vi "Str To Colorbox.vi"(1 "String":string) -> (0 "Color Box":u32(colorbox))   [LabVIEW 2017]
doc: "Converts a colour string into the 32-bit RGB value that a LabVIEW colour box control displays."
uses:
  _openG/_reuse_openG.lvlib
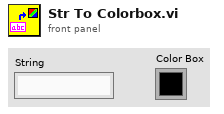
[diagram p1: front panel]
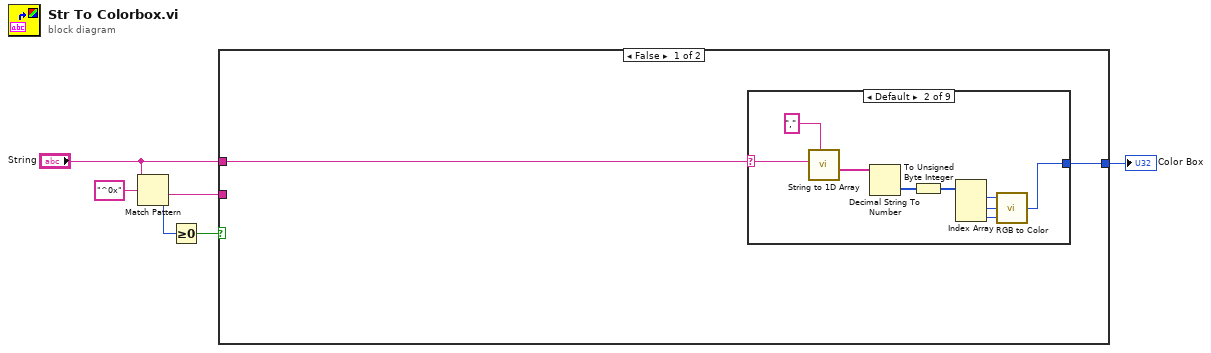
[diagram p0: block diagram]
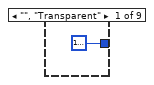
[diagram p2: hidden frame]
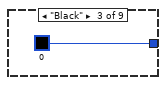
[diagram p3: hidden frame]
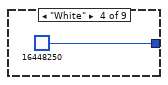
[diagram p4: hidden frame]
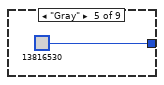
[diagram p5: hidden frame]
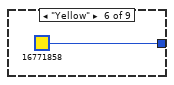
[diagram p6: hidden frame]
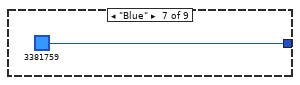
[diagram p7: hidden frame]
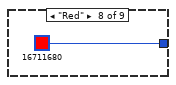
[diagram p8: hidden frame]
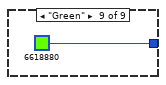
[diagram p9: hidden frame]
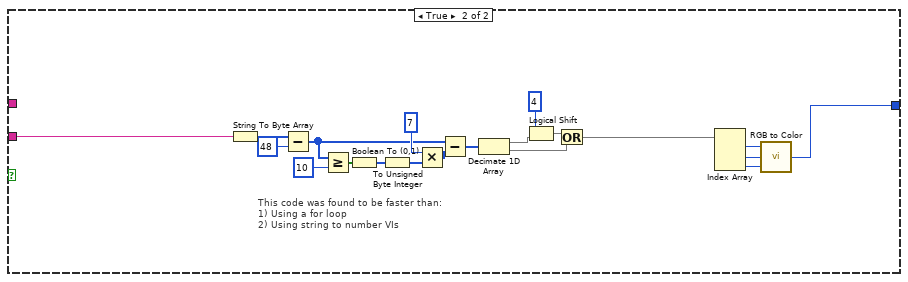
[diagram p10: hidden frame]
diagram:
  n1 = Match Pattern(string="String", regular expression="^0x") -> (after substring=w1:string, offset past match=w3:i32)  [unwired: 1 in, 2 out]
  n2 = Greater Or Equal To 0?(x=w3) -> (x >= 0?=w2:bool)
  n3 = case shown="False" w2 {
    tunnel: [w8 w40] -> w6
    tunnel: "String" -> [w7 _]
    tunnel: w1 -> [_ w45]
    frame False {
      n4 = case shown="Default" w7 {
        selector: w7 -> [_ w14 _ _ _ _ _ _ _]
        tunnel: [u32 16777216 w13 u32 0 u32 16448250 u32 13816530 u32 16771858 u32 3381759 u32 16711680 u32 6618880] -> w8
        frame "", "Transparent" {
        }
        frame Default {
          n5 = call "String to 1D Array.vi"("delimiter (Tab)"=",", "string"=w14) -> ("Array of Strings"=w18:string[])  [unwired: 9 in]
          n6 = Decimal String To Number(string=w18) -> (number=w11:i32[])  [unwired: 2 in, 1 out]
          n7 = To Unsigned Byte Integer(number=w11) -> (unsigned 8bit integer=w10:u8[])
          n8 = Index Array(array=w10) -> (element #1=w17:u8, element #2=w16:u8, element #3=w15:u8)  [unwired: 3 in]
          n9 = call <vilib>:"RGB to Color.vi"("B"=w15, "G"=w16, "R"=w17) -> ("Color"=w13:u32)
        }
        frame "Black" {
        }
        frame "White" {
        }
        frame "Gray" {
        }
        frame "Yellow" {
        }
        frame "Blue" {
        }
        frame "Red" {
        }
        frame "Green" {
        }
      }
    }
    frame True {
      # "This code was found to be faster than:\n1) Using a for loop\n2) Using string to number VIs"
      n10 = String To Byte Array(string=w45) -> (unsigned byte array=w39:u8[])
      n11 = Subtract(x=w39, y=u8 48) -> (x-y=w28:u8[])
      n12 = Greater Or Equal?(x=w28, y=u8 10) -> (x >= y?=w31:bool[])
      n13 = Boolean To (0,1)(Boolean=w31) -> (0, 1=w33:i16[])
      n14 = To Unsigned Byte Integer(number=w33) -> (unsigned 8bit integer=w30:u8[])
      n15 = Multiply(x=u8 7, y=w30) -> (x*y=w29:u8[])
      n16 = Subtract(x=w28, y=w29) -> (x-y=w37:u8[])
      n17 = Decimate 1D Array(w37) -> (w36:u8[], w38:u8[])
      n18 = Logical Shift(y=i8 4, x=w36) -> (x << y=w27:u8[])
      n19 = Or(x=w27, y=w38) -> (x .or. y?=w44:u8[])
      n20 = Index Array(array=w44) -> (element #1=w43:u8, element #2=w42:u8, element #3=w41:u8)  [unwired: 3 in]
      n21 = call <vilib>:"RGB to Color.vi"("B"=w41, "G"=w42, "R"=w43) -> ("Color"=w40:u32)
    }
  }
  "Color Box" <- w6
